vi "v_piezo_scaling.vi"(5 "Stack commands (nominal microns)":sgl[](array[numeric])) -> (1 "DAC out (volts)":sgl[](array[numeric]))   [LabVIEW 2010]
panel:
  in  "V min":sgl=-10.0
  in  "V max":sgl=120.0
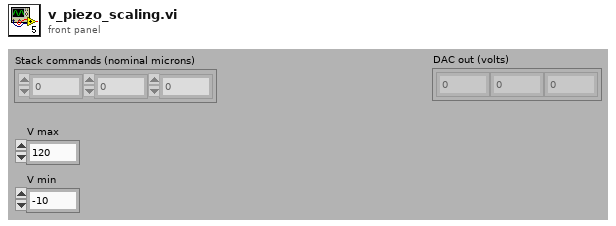
[diagram p1: front panel]
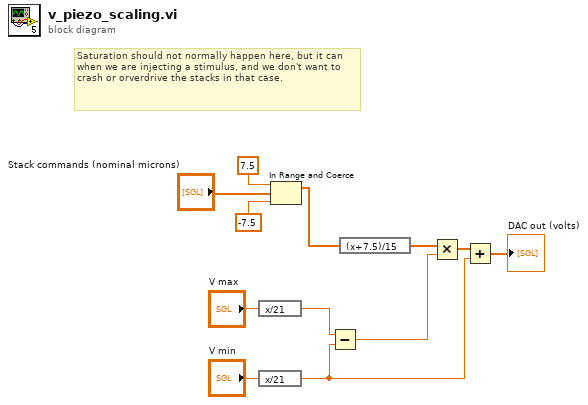
[diagram p0: block diagram]
diagram:
  # "Saturation should not normally happen here, but it can when we are injecting a stimulus, and we don't want to crash or orverdrive the stacks in that case."
  n1 = expression code="x/21"("V max") -> (w10:sgl)
  n2 = expression code="x/21"("V min") -> (w6:sgl)
  n3 = In Range and Coerce(upper limit=sgl 7.5, x="Stack commands (nominal microns)", lower limit=sgl -7.5) -> (coerced(x)=w2:sgl[])  [unwired: 1 out]
  n4 = Subtract(x=w10, y=w6) -> (x-y=w8:sgl)
  n5 = expression code="(x+7.5)/15"(w2) -> (w9:sgl[])
  n6 = Multiply(x=w9, y=w8) -> (x*y=w7:sgl[])
  n7 = Add(x=w7, y=w6) -> (x+y=→"DAC out (volts)":sgl[])
